vi "WriteAlarmRules.vi"(8 "error in (no error)":errorcluster, 11 "alarm rules":T1[](array[typedef])) -> (0 "error out":errorcluster)   [LabVIEW 2017, in "ServerComm.lvlib"]
uses:
  <vilib>/addons/InsightCM/Devices/Shared/Common/ServerComm/ServerComm.lvlib
  <vilib>/addons/InsightCM/MessageBus/Base/controls/AlarmRule.ctl
  <vilib>/addons/InsightCM/MessageBus/Base/controls/AlarmTrigger.ctl
  <vilib>/addons/InsightCM/MessageBus/Base/controls/AlarmCondition.ctl
  <vilib>/addons/InsightCM/MessageBus/Base/controls/AlarmAction.ctl
  <vilib>/addons/InsightCM/MessageBus/Base/controls/KeyValuePair.ctl
  <vilib>/addons/InsightCM/Utilities/GlobalConfiguration/GlobalConfiguration.lvlib
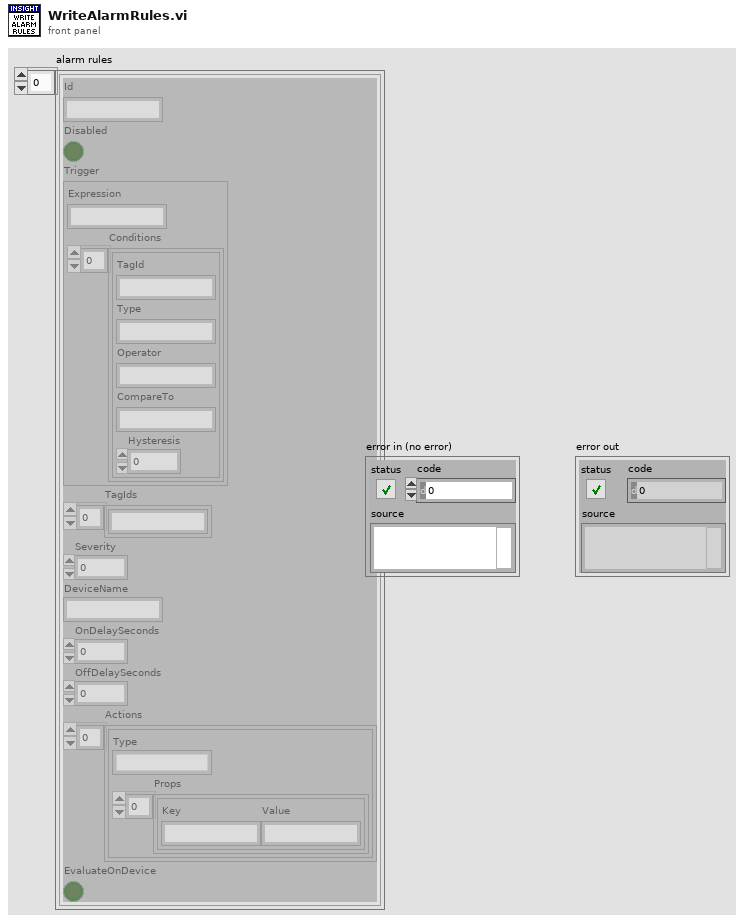
[diagram p1: front panel]
types:
  T1 = typedef "AlarmRule.ctl" = cluster{"Id":string, "Disabled":bool, "Trigger":T2, "TagIds":string[], "Severity":i32, "DeviceName":string, "OnDelaySeconds":dbl, "OffDelaySeconds":dbl, "Actions":T4[], "EvaluateOnDevice":bool}
  T2 = typedef "AlarmTrigger.ctl" = cluster{"Expression":string, "Conditions":T3[]}
  T3 = typedef "AlarmCondition.ctl" = cluster{"TagId":string, "Type":string, "Operator":string, "CompareTo":string, "Hysteresis":dbl}
  T4 = typedef "AlarmAction.ctl" = cluster{"Type":string, "Props":T5[]}
  T5 = typedef "KeyValuePair.ctl" = cluster{"Key":string, "Value":string}
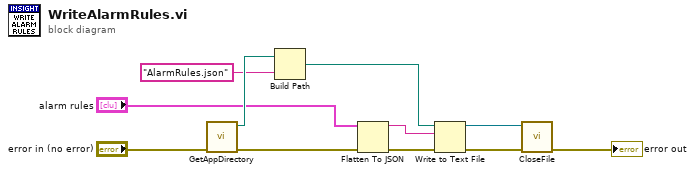
[diagram p0: block diagram]
diagram:
  n1 = call <vilib>:"GetAppDirectory.vi"("error in (no error)"="error in (no error)") -> ("error out"=w8:errorcluster, "application directory"=w10:path)  [unwired: 9 in]
  n2 = Build Path(base path=w10, name or relative path="AlarmRules.json") -> (appended path=w5:path)
  n3 = Flatten To JSON(anything="alarm rules", error in (no error)=w8) -> (JSON string=w4:string, 11:w7:errorcluster)  [unwired: 1 in]
  n4 = Write to Text File(file (use dialog)=w5, text=w4, error in=w7) -> (refnum out=w3:refnum<file>, error out=w1:errorcluster)  [unwired: 1 in, 1 out]
  n5 = call <vilib>:"CloseFile.vi"("error in (no error)"=w1, "file reference"=w3) -> ("error out"=→"error out":errorcluster)  [unwired: 9 in]
